vi "Hight_control.vi"(7 "Á³±ì°ª«×":dbl(ring)=300.0 items=["物料櫃第一格"=0.0, "物料櫃第二格"=85.0, "Á³´U§¨¨ú°ª«×"=128.0, "Á³´UºË·Ç"=250.0, "最高"=288.0], 8 "Error In":errorcluster) -> (0 "Error Out":errorcluster)   [LabVIEW 2019]
uses:
  WSCbot_V3_Toolkit.lvlibp
panel:
  out "PresentPOS":dbl
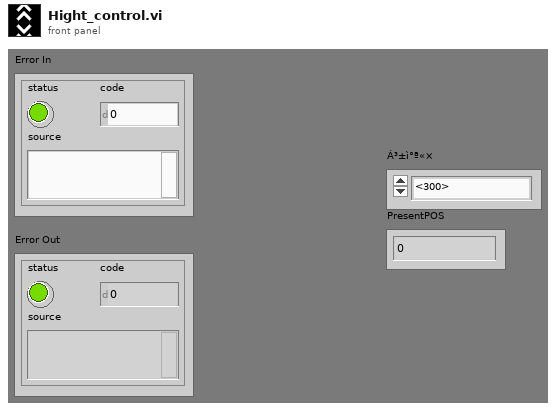
[diagram p1: front panel]
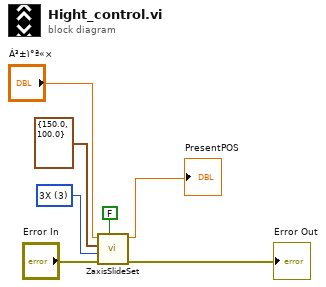
[diagram p0: block diagram]
diagram:
  w5 = u16 3 items=["0X", "1X", "2X", "3X"] ("findHomeVel (times)")
  n1 = call "ZaxisSlideSet.vi"("Reset"=FALSE, "error in"="Error In", "findHomeVel (times)"=w5, "Velocity(mm/s)&ACC(mm/ss)"=cluster{"Velocity(cm/s)":dbl, "ACC(cm/ss)":dbl} {"Velocity(cm/s)"=150.0, "ACC(cm/ss)"=100.0}, "TargetABSHight(mm)"="Á³±ì°ª«×") -> ("error out"=→"Error Out":errorcluster, "PresentPOS(mm)"=→"PresentPOS":dbl)  [unwired: 5 in]
